vi "GetAMIRequest.vi"(10 "Address":u8=1, 11 "Checksum used":bool=TRUE) -> (3 "Request":string)   [LabVIEW 2017]
uses:
  <instrlib>/Samwontech TEMP2xxx/Samwontech TEMP2xxx.lvlib
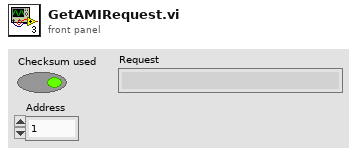
[diagram p1: front panel]
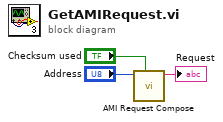
[diagram p0: block diagram]
diagram:
  n1 = call <instrlib>:"AMI Request Compose.vi"("Checksum used"="Checksum used", "Address"="Address") -> ("Request"=→"Request":string)  [unwired: 8 in, 1 out]
